vi "Initialize.vi"(5 "Custom Device in":refnum<class "Custom Device.lvclass">, 7 "Custom Device Name":string, 8 "error in":errorcluster, 9 "Compiled Settings":variant, 10 "Custom Device API in":refnum<class "Custom Device API.lvclass">) -> (0 "error out":errorcluster, 3 "Custom Device Utility out":refnum<class "Custom Device Utility.lvclass">)   [LabVIEW 2027, in "Custom Device Interfaces.lvlib" / "Custom Device Utility.lvclass"]
uses:
  Custom Device Utility.lvclass
  CustomDeviceAPI/Custom Device API.lvclass
  CustomDevice/Custom Device.lvclass
  Custom Device Utility.lvclass/Custom Device Utility.ctl
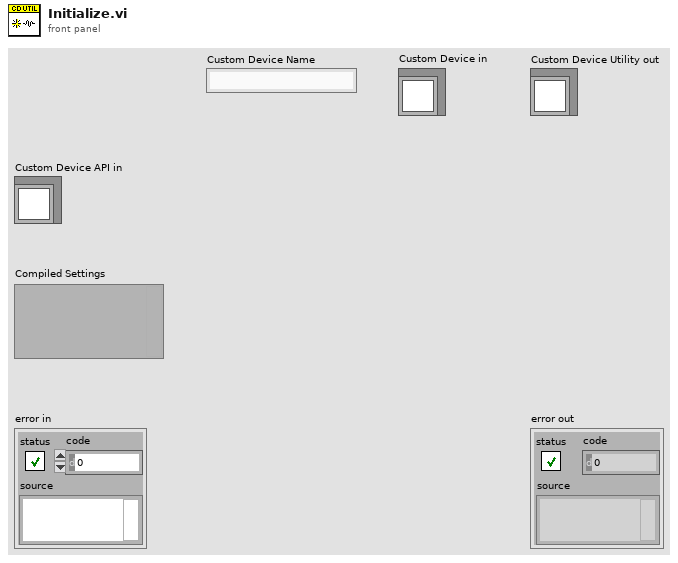
[diagram p1: front panel]
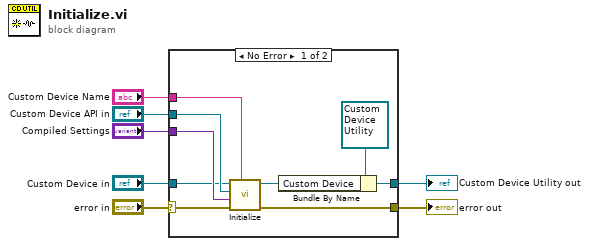
[diagram p0: block diagram]
diagram:
  n1 = case shown="No Error" "error in" {
    selector: "error in" -> [w11 w17]
    tunnel: [w16 w17] -> w6
    tunnel: [w15 _] -> w1
    tunnel: "Custom Device API in" -> [w14 _]
    tunnel: "Compiled Settings" -> [w13 _]
    tunnel: "Custom Device Name" -> [w12 _]
    tunnel: "Custom Device in" -> [w10 _]
    frame No Error {
      n2 = call-dynamic "Initialize.vi"("Custom Device Name"=w12, "error in"=w11, "Compiled Settings"=w13, "Custom Device API in"=w14, "Custom Device In"=w10) -> ("error out"=w16:errorcluster, "Custom Device out"=w9:refnum<class "Custom Device.lvclass">)  [unwired: 5 in]
      n3 = Bundle By Name(cluster=refnum<class "Custom Device Utility.lvclass"> refnum ("CustomDeviceInterfaces.lvlib:CustomDeviceUtility.lvclass"), "Custom Device"=w9) -> (w15:refnum<class "Custom Device Utility.lvclass">)
    }
    frame Error {
    }
  }
  "error out" <- w6
  "Custom Device Utility out" <- w1
